vi "VCI_GetReference2.vi"(8 "error in (no error)":errorcluster caption="错误输入（无错误）", 9 "CANIndex":u32, 10 "DevIndex":u32, 11 "DevType":T14=2 items=["USB-CAN"=2, "USB-CAN2"=3]) -> (0 "error out":errorcluster caption="错误输出", 2 "RefStruct":T1={"RefNormal"={"Mode"=0, "Fliter"=1, "AccCode"=0, "AccMask"=0, "kBaudRate"=0, "Timing0"=0, "Timing1"=0, "CANRX_EN"=0, "UARTBAUD"=0}, "Reserved"=0, "BaudType"={"Baud"=0, "SJW"=1, "BRP"=1, "SAM"=0, "PHSEG2_SEL"=0, "PRSEG"=1, "PHSEG1"=1, "PHSEG2"=1}} {"RefNormal"."kBaudRate" items=["SelfDefine", "5 kbps", "10 kbps", "20 kbps", "40 kbps", "50 kbps", "80 kbps", "100 kbps", "125 kbps", "200 kbps", "250 kbps", "400 kbps", "500 kbps", "666 kbps", "800 kbps", "1000 kbps", "33.33 kbps", "66.66 kbps", "83.33 kbps"]; "RefNormal"."AccMask" format="%x"; "RefNormal"."AccCode" format="%x"; "RefNormal"."Fliter" items=["接收所有类型"=1, "只接收标准帧"=2, "只接收扩展帧"=3]; "RefNormal"."Mode" items=["正常工作", "仅侦听模式", "自测模式（环回）"]; "BaudType"."PHSEG2" items=["CAN_BIT_1TQ"=1, "CAN_BIT_2TQ"=2, "CAN_BIT_3TQ"=3, "CAN_BIT_4TQ"=4, "CAN_BIT_5TQ"=5, "CAN_BIT_6TQ"=6, "CAN_BIT_7TQ"=7, "CAN_BIT_8TQ"=8]; "BaudType"."PHSEG1" items=["CAN_BIT_1TQ"=1, "CAN_BIT_2TQ"=2, "CAN_BIT_3TQ"=3, "CAN_BIT_4TQ"=4, "CAN_BIT_5TQ"=5, "CAN_BIT_6TQ"=6, "CAN_BIT_7TQ"=7, "CAN_BIT_8TQ"=8]; "BaudType"."PRSEG" items=["CAN_BIT_1TQ"=1, "CAN_BIT_2TQ"=2, "CAN_BIT_3TQ"=3, "CAN_BIT_4TQ"=4, "CAN_BIT_5TQ"=5, "CAN_BIT_6TQ"=6, "CAN_BIT_7TQ"=7, "CAN_BIT_8TQ"=8]; "BaudType"."PHSEG2_SEL" items=["由相位缓冲段1时间决定", "可编程"]; "BaudType"."SAM" items=["采样一次", "采样三次"]; "BaudType"."BRP" items=["1"=1, "2"=2, "3"=3, "4"=4, "5"=5, "6"=6, "7"=7, "8"=8, "9"=9, "10"=10, "11"=11, "12"=12, "13"=13, "14"=14, "15"=15, "16"=16, "17"=17, "18"=18, "19"=19, "20"=20, "21"=21, "22"=22, "23"=23, "24"=24, "25"=25, "26"=26, "27"=27, "28"=28, "29"=29, "30"=30, "31"=31, "32"=32, "33"=33, "34"=34, "35"=35, "36"=36, "37"=37, "38"=38, "39"=39, "40"=40, "41"=41, "42"=42, "43"=43, "44"=44, "45"=45, "46"=46, "47"=47, "48"=48, "49"=49, "50"=50, "51"=51, "52"=52, "53"=53, "54"=54, "55"=55, "56"=56, "57"=57, "58"=58, "59"=59, "60"=60, "61"=61, "62"=62, "63"=63, "64"=64]; "BaudType"."SJW" items=["1TQ"=1, "2TQ"=2, "3TQ"=3, "4TQ"=4]}, 3 "Return Val":T15=1 items=["OK"=1, "ERROR1"=0, "ERROR2"=-1])   [LabVIEW 2018, in "ControlCan.lvlib"]
uses:
  ControlCan.lvlib
  Return Val.ctl
  DevType.ctl
  RefStruct.ctl
  RefNormal.ctl
  Mode.ctl
  Fliter.ctl
  kBaudRate.ctl
  BaudType.ctl
  SJW.ctl
  BRP.ctl
  SAM.ctl
  PHSEG2_SEL.ctl
  PRSEG.ctl
  PHSEG1.ctl
  PHSEG2.ctl
  RefStruct_1.ctl
panel:
  in  "pTempBuff":u8[](array[numeric])
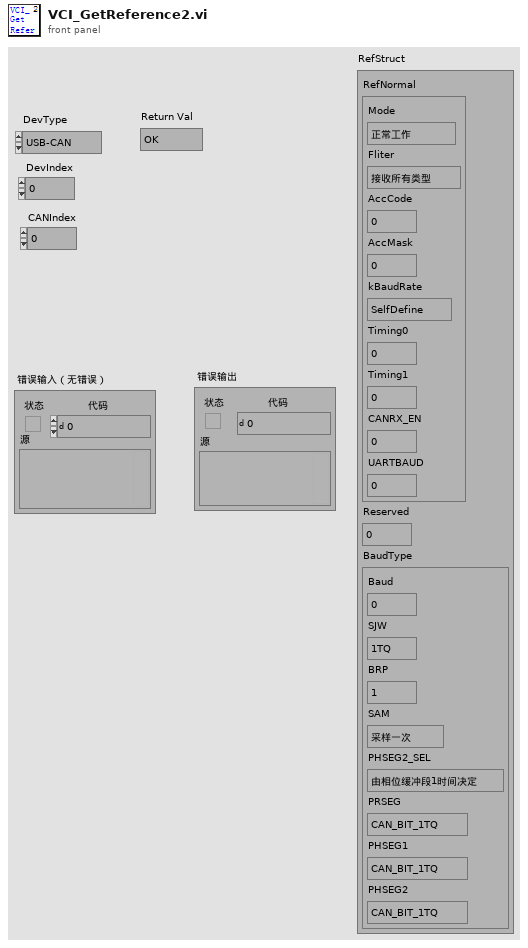
[diagram p1: front panel]
types:
  T1 = typedef "ControlCAN.lvlib/RefStruct.ctl" = cluster{"RefNormal":T2, "Reserved":u8, "BaudType":T6}
  T2 = typedef "ControlCAN.lvlib/RefNormal.ctl" = cluster{"Mode":T3, "Fliter":T4, "AccCode":u32, "AccMask":u32, "kBaudRate":T5, "Timing0":u8, "Timing1":u8, "CANRX_EN":u8, "UARTBAUD":u8}
  T3 = typedef "ControlCAN.lvlib/Mode.ctl" = u8
  T4 = typedef "ControlCAN.lvlib/Fliter.ctl" = u8
  T5 = typedef "ControlCAN.lvlib/kBaudRate.ctl" = u8
  T6 = typedef "ControlCAN.lvlib/BaudType.ctl" = cluster{"Baud":u32, "SJW":T7, "BRP":T8, "SAM":T9, "PHSEG2_SEL":T10, "PRSEG":T11, "PHSEG1":T12, "PHSEG2":T13}
  T7 = typedef "ControlCAN.lvlib/SJW.ctl" = u8
  T8 = typedef "ControlCAN.lvlib/BRP.ctl" = u8
  T9 = typedef "ControlCAN.lvlib/SAM.ctl" = u8
  T10 = typedef "ControlCAN.lvlib/PHSEG2_SEL.ctl" = u8
  T11 = typedef "ControlCAN.lvlib/PRSEG.ctl" = u8
  T12 = typedef "ControlCAN.lvlib/PHSEG1.ctl" = u8
  T13 = typedef "ControlCAN.lvlib/PHSEG2.ctl" = u8
  T14 = typedef "ControlCAN.lvlib/DevType.ctl" = u32
  T15 = typedef "ControlCAN.lvlib/Return Val.ctl" = i32
  T16 = typedef "ControlCAN.lvlib/RefStruct_1.ctl" = cluster{"Mode":T3, "Fliter":T4, "ACR 0":u8, "ACR 1":u8, "ACR 2":u8, "ACR 3":u8, "AMR 0":u8, "AMR 1":u8, "AMR 2":u8, "AMR 3":u8, "kBaudRate":T5, "Timing 0":u8, "Timing 1":u8, "CANRX_EN":u8, "UARTBAUD":u8, "Reserved":u8, "Baud 0":u8, "Baud 1":u8, "Baud 2":u8, "Baud 3":u8, "SJW":T7, "BRP":T8, "SAM":T9, "PHSEG2_SEL":T10, "PRSEG":T11, "PHSEG1":T12, "PHSEG2":T13}
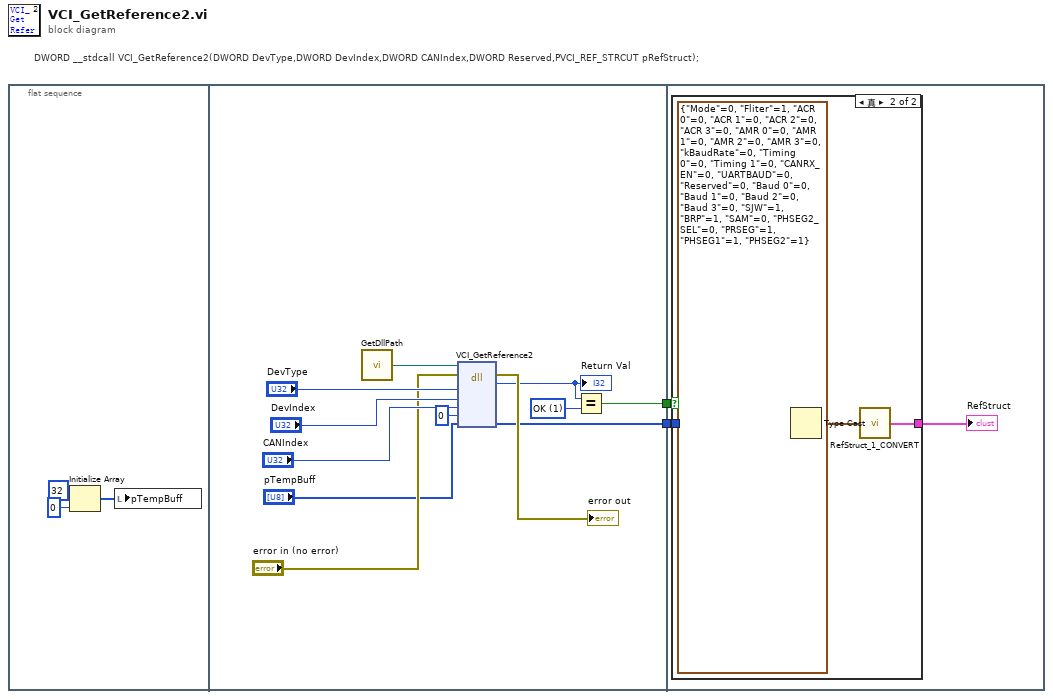
[diagram p0: block diagram]
diagram:
  # "DWORD __stdcall VCI_GetReference2(DWORD DevType,DWORD DevIndex,DWORD CANIndex,DWORD Reserved,PVCI_REF_STRCUT pRefStruct);"
  n1 = flat-sequence {
    tunnel: [w8] -> w2
    tunnel: [w7] -> w1
    tunnel: w2 -> [w20]
    tunnel: w1 -> [w19]
    frame #0 {
      n2 = Initialize Array(u8 32, 0 ("维数大小")) -> (w3:u8[])
      n3 = local write "pTempBuff"(w3) -> ()
    }
    frame #1 {
      w9 = T15 1 items=["OK"=1, "ERROR1"=0, "ERROR2"=-1] ("Return Val")
      n4 = call "GetDllPath.vi"() -> ("DllPath"=w6:path)  [unwired: 1 in]
      n5 = dll-call lib="?" fn="VCI_GetReference2"(path in=w6, error in="error in (no error)", "DevType"="DevType", "DevIndex"="DevIndex", "CANIndex"="CANIndex", "Reserved"=u32 0, "pRefStruct"="pTempBuff") -> (error out=→"error out":errorcluster, "ReturnVal"=w10:i32, "pRefStruct"=w7:u8[])  [unwired: 5 in, 1 out]
      "Return Val" <- w10
      n6 = Equal?(x=w10, y=w9) -> (x = y?=w8:bool)
    }
    frame #2 {
      n7 = case shown="真" w20 {
        tunnel: w19 -> [_ w23]
        tunnel: [_ w21] -> w18
        frame False {
        }
        frame True {
          n8 = Type Cast(type=T16 {"Mode"=0, "Fliter"=1, "ACR 0"=0, "ACR 1"=0, "ACR 2"=0, "ACR 3"=0, "AMR 0"=0, "AMR 1"=0, "AMR 2"=0, "AMR 3"=0, "kBaudRate"=0, "Timing 0"=0, "Timing 1"=0, "CANRX_EN"=0, "UARTBAUD"=0, "Reserved"=0, "Baud 0"=0, "Baud 1"=0, "Baud 2"=0, "Baud 3"=0, "SJW"=1, "BRP"=1, "SAM"=0, "PHSEG2_SEL"=0, "PRSEG"=1, "PHSEG1"=1, "PHSEG2"=1} ("RefStruct_1"), x=w23) -> (*(type *) &x=w22:T16)
          n9 = call "RefStruct_1_CONVERT.vi"("RefStruct_1"=w22) -> ("RefStruct"=w21:T1)
        }
      }
      "RefStruct" <- w18
    }
  }
